vi "Table handling DEBUG.vi"() -> ()   [LabVIEW 2013]
panel:
  in  "Calibration Details":string[][](table)=[["Calibrator Name", "Procedure", "Calibration Interval", "Date Complete", "Date Due", "Calibrator Signature"]]
  in  "Instrument Identification":string[][](table)=[["Gauge Number:"], ["Common Identifier:"], ["Manufacturer:"], ["Model Number:"], ["Description:"], ["Serial Number:"], ["In-Service Date:"], ["Condition:"]]
  in  "Environment Details":string[][](table)=[["Company:", "TI Automotive"], ["Building:", "Caro Test Center"], ["Street Address:", "628 Columbia St."], ["City Address:", "Caro, MI 48723"], ["Room Name:", ""], ["Room Temperature:", ""], ["Room Humidity:", ""]]
  in  "Standards Used":string[][](table)=[["Description:", "Gauge Number:", "Units:", "Unit Abbreviation:", "Calibration Due:"]]
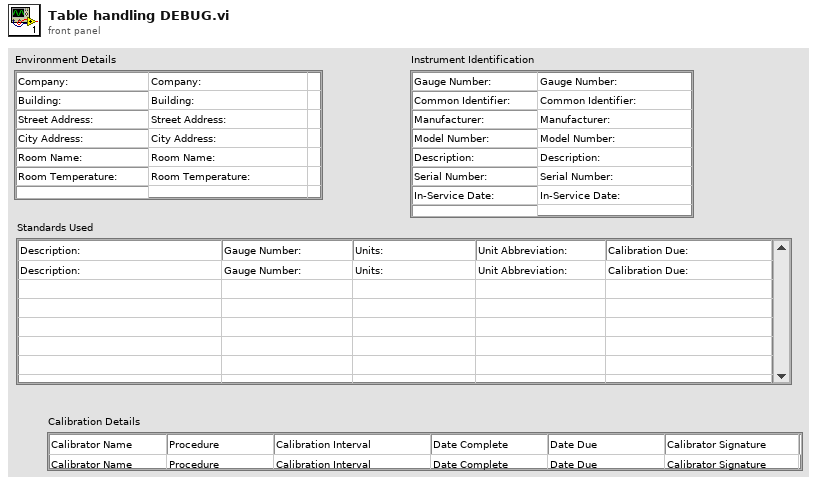
[diagram p1: front panel]
types:
  T1 = typedef "eventvkey.ctl" = enum16{"ASCII", "Enter", "Return", "Shift", "Ctrl", "Alt", "Cmd", "Opt", "Caps", "NumLock", "Clear", "Break", "Up", "Down", "Left", "Right", "Insert", "Delete", "Home", "End", "PageUp", "PageDown", "Escape", "Help", "Pause", "ScrollLock", "F1", "F2", "F3", "F4", "F5", "F6", "F7", "F8", "F9", "F10", "F11", "F12", "F13", "F14", "F15", "F16", "F17", "F18", "F19", "F20", "F21", "F22", "F23", "F24", "Play", "VolumeUp", "VolumeDown", "Mute", "Two Byte Char"}
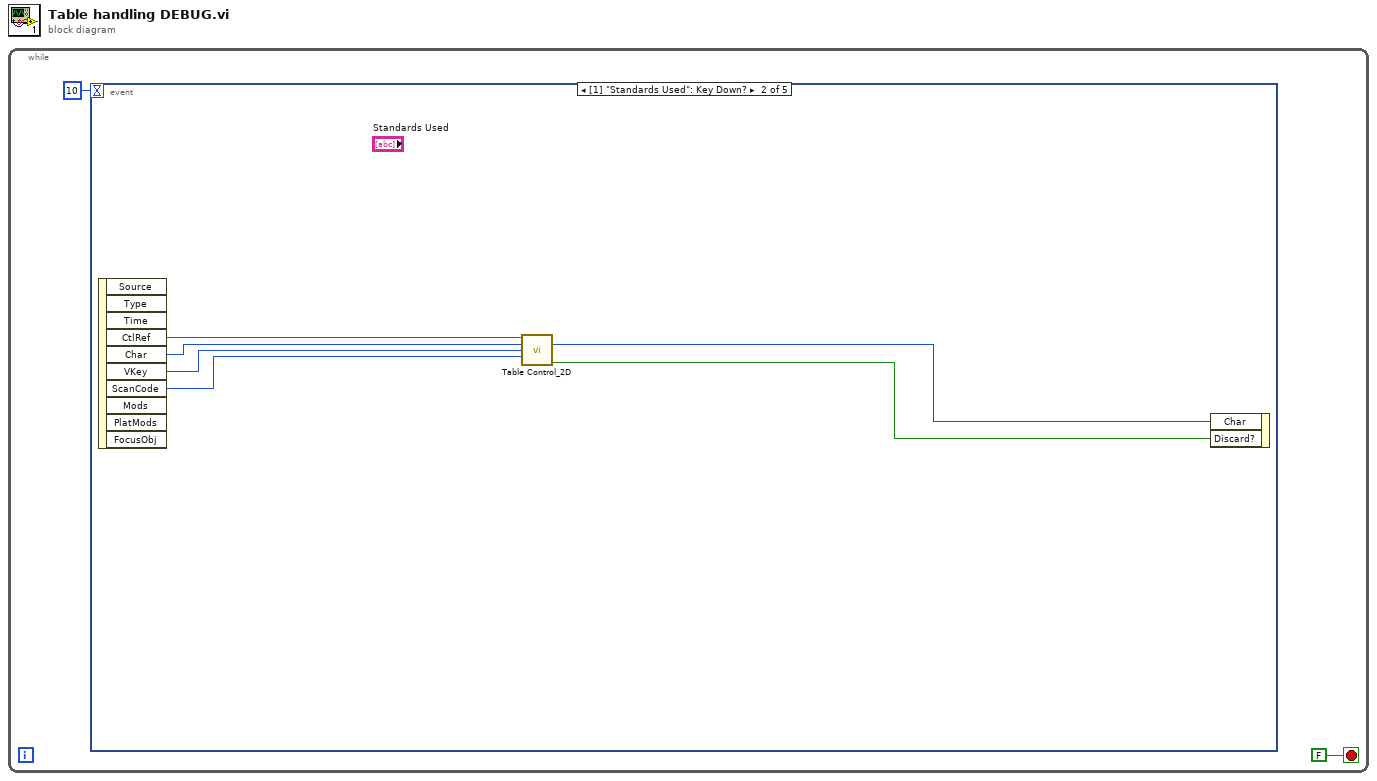
[diagram p0: block diagram]
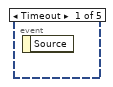
[diagram p2: hidden frame]
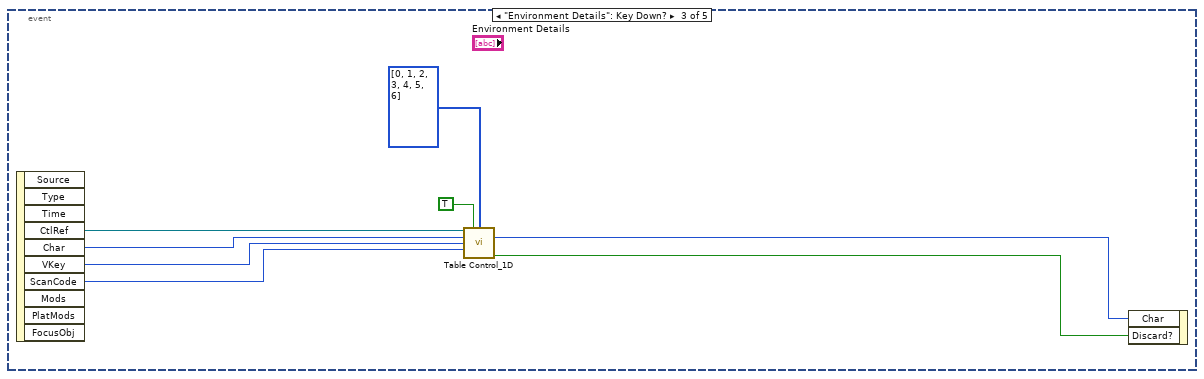
[diagram p3: hidden frame]
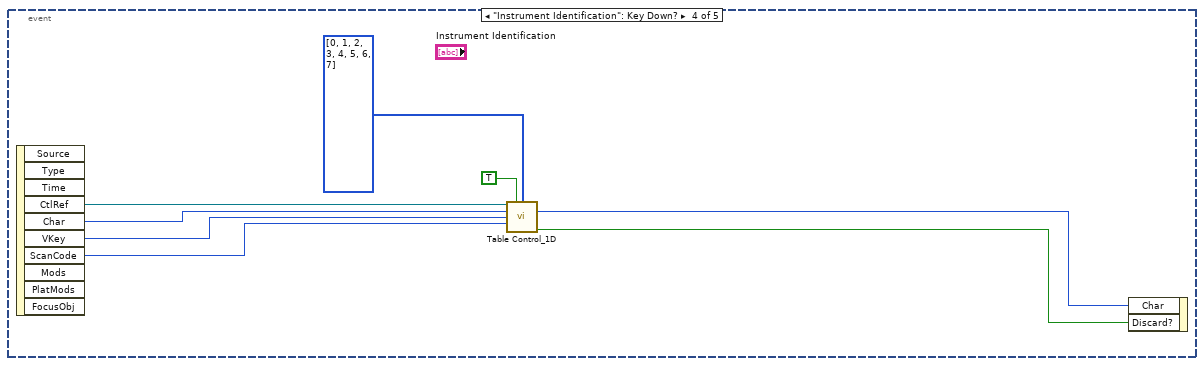
[diagram p4: hidden frame]
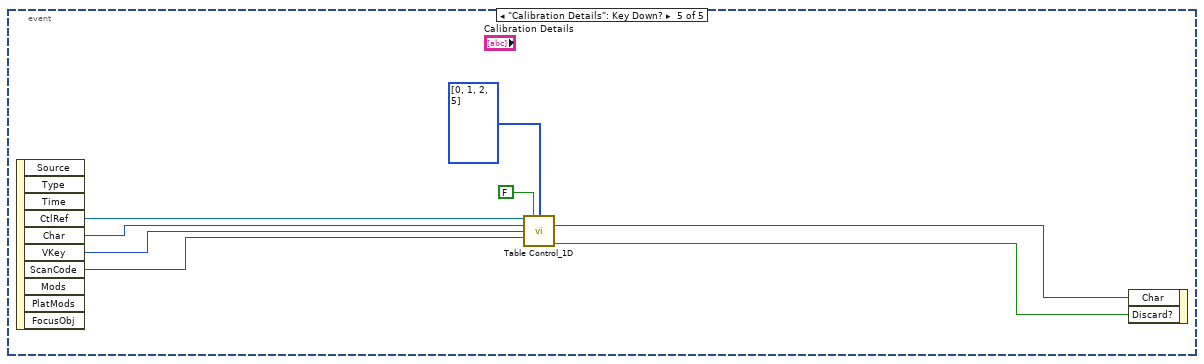
[diagram p5: hidden frame]
diagram:
  n1 = while {
    stop <- FALSE stop-if-true
    n2 = event shown="[1] \"Standards Used\": Key Down?" {
      selector: _ -> [_ _ _ _ _]
      dyn-events: _ -> [_ _ _ _ _]
      timeout: 10 -> [_ _ _ _ _]
      event Timeout {
        n3 = event-data() -> ()  [unwired: 1 in, 1 out]
      }
      event "Standards Used": Key Down? {
        n4 = event-data() -> ("CtlRef"=w8:refnum<vi>, "Char"=w7:i16, "VKey"=w4:T1, "ScanCode"=w3:i16)  [unwired: 1 in, 6 out]
        n5 = call "Table Control_2D.vi"("CtlRef"=w8, "CharIn"=w7, "VKey"=w4, "ScanCode"=w3) -> ("CharOut"=w6:i16, "Discard?"=w5:bool)  [unwired: 10 in]
        n6 = event-data("Char"=w6, "Discard?"=w5) -> ()  [unwired: 1 in, 1 out]
      }
      event "Environment Details": Key Down? {
        n7 = event-data() -> ("CtlRef"=w16:refnum<vi>, "Char"=w15:i16, "VKey"=w14:T1, "ScanCode"=w13:i16)  [unwired: 1 in, 6 out]
        n8 = call "Table Control_1D.vi"("CtlRef"=w16, "Header Row(F)/Column(T)"=TRUE, "Valid Indexes"=i32[] [0, 1, 2, 3, 4, 5, 6], "CharIn"=w15, "VKey"=w14, "ScanCode"=w13) -> ("CharOut"=w12:i16, "Discard?"=w11:bool)  [unwired: 8 in]
        n9 = event-data("Char"=w12, "Discard?"=w11) -> ()  [unwired: 1 in, 1 out]
      }
      event "Instrument Identification": Key Down? {
        n10 = event-data() -> ("CtlRef"=w22:refnum<vi>, "Char"=w21:i16, "VKey"=w20:T1, "ScanCode"=w19:i16)  [unwired: 1 in, 6 out]
        n11 = call "Table Control_1D.vi"("CtlRef"=w22, "Header Row(F)/Column(T)"=TRUE, "Valid Indexes"=i32[] [0, 1, 2, 3, 4, 5, 6, 7], "CharIn"=w21, "VKey"=w20, "ScanCode"=w19) -> ("CharOut"=w23:i16, "Discard?"=w24:bool)  [unwired: 8 in]
        n12 = event-data("Char"=w23, "Discard?"=w24) -> ()  [unwired: 1 in, 1 out]
      }
      event "Calibration Details": Key Down? {
        n13 = event-data() -> ("CtlRef"=w32:refnum<vi>, "Char"=w31:i16, "VKey"=w30:T1, "ScanCode"=w29:i16)  [unwired: 1 in, 6 out]
        n14 = call "Table Control_1D.vi"("CtlRef"=w32, "Header Row(F)/Column(T)"=FALSE, "Valid Indexes"=i32[] [0, 1, 2, 5], "CharIn"=w31, "VKey"=w30, "ScanCode"=w29) -> ("CharOut"=w27:i16, "Discard?"=w28:bool)  [unwired: 8 in]
        n15 = event-data("Char"=w27, "Discard?"=w28) -> ()  [unwired: 1 in, 1 out]
      }
    }
  }
